vi "k2DInterp.vi"(8 "col":dbl, 9 "row":dbl, 11 "Array":dbl[][](array[numeric])) -> (3 "result":dbl)   [LabVIEW 2016, in "KevLib01.lvlib"]
uses:
  KevLib01.lvlib
panel:
  # "Note: Index works as a normal index will, ie (3,5) will return the (3,5) element in the array."
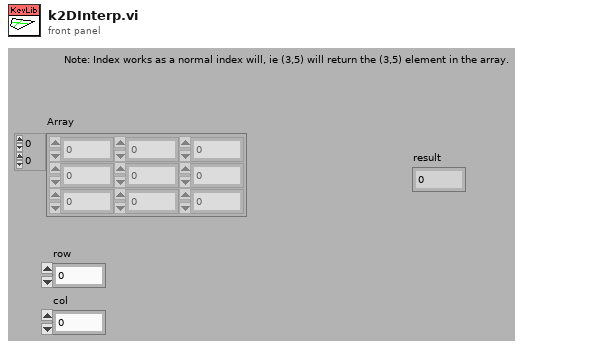
[diagram p1: front panel]
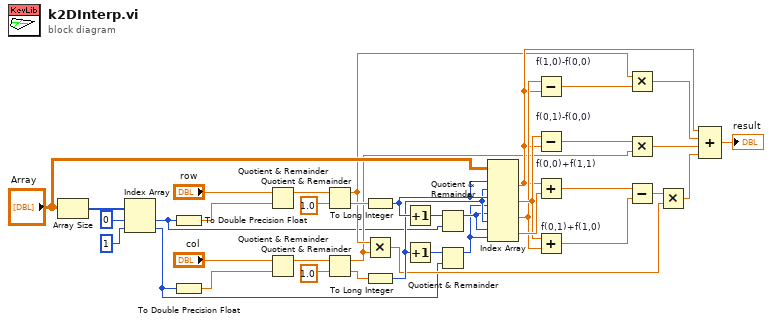
[diagram p0: block diagram]
diagram:
  n1 = Array Size(array="Array") -> (size(s)=w38:i32[])
  n2 = Index Array(array=w38, index #1=0 ("index"), index #2=1 ("index")) -> (element #1=w7:i32, element #2=w4:i32)
  n3 = To Double Precision Float(number=w7) -> (double precision float=w35:dbl)
  n4 = To Double Precision Float(number=w4) -> (double precision float=w34:dbl)
  n5 = Quotient & Remainder(x="row", y=w35) -> (x-y*floor(x/y)=w30:dbl)  [unwired: 1 out]
  n6 = Quotient & Remainder(x="col", y=w34) -> (x-y*floor(x/y)=w27:dbl)  [unwired: 1 out]
  n7 = Quotient & Remainder(x=w30, y=1.0) -> (x-y*floor(x/y)=w16:dbl, floor(x/y)=w25:dbl)
  n8 = Quotient & Remainder(x=w27, y=1.0) -> (x-y*floor(x/y)=w15:dbl, floor(x/y)=w26:dbl)
  n9 = To Long Integer(number=w25) -> (32bit integer=w32:i32)
  n10 = Multiply(x=w16, y=w15) -> (x*y=w14:dbl)
  n11 = To Long Integer(number=w26) -> (32bit integer=w31:i32)
  n12 = Increment(x=w32) -> (x+1=w8:i32)
  n13 = Increment(x=w31) -> (x+1=w5:i32)
  n14 = Quotient & Remainder(x=w8, y=w7) -> (x-y*floor(x/y)=w6:i32)  [unwired: 1 out]
  n15 = Quotient & Remainder(x=w5, y=w4) -> (x-y*floor(x/y)=w3:i32)  [unwired: 1 out]
  n16 = Index Array(array="Array", index (row) #1=w32, index (col) #1=w31, index (row) #2=w32, index (col) #2=w3, index (row) #3=w6, index (col) #3=w31, index (row) #4=w6, index (col) #4=w3) -> (element #1=w19:dbl, element #2=w23:dbl, element #3=w22:dbl, element #4=w24:dbl)
  n17 = Subtract "f(1,0)-f(0,0)"(x=w22, y=w19) -> (x-y=w18:dbl)
  n18 = Subtract "f(0,1)-f(0,0)"(x=w23, y=w19) -> (x-y=w17:dbl)
  n19 = Add "f(0,0)+f(1,1)"(x=w19, y=w24) -> (x+y=w21:dbl)
  n20 = Add "f(0,1)+f(1,0)"(x=w23, y=w22) -> (x+y=w20:dbl)
  n21 = Multiply(x=w16, y=w18) -> (x*y=w10:dbl)
  n22 = Multiply(x=w17, y=w15) -> (x*y=w11:dbl)
  n23 = Subtract(x=w21, y=w20) -> (x-y=w13:dbl)
  n24 = Multiply(x=w13, y=w14) -> (x*y=w12:dbl)
  n25 = Compound Arithmetic op=ADD(w19, w10, w11, w12) -> (→"result":dbl)
